vi "PKG_IMC_ClearIMC.vi"(11 "handle":u32) -> (2 "function return":i32, 3 "handle out":u32)   [LabVIEW 2018, in "IMC_Pkg4xxx.lvlib"]
doc: "PKG_IMC_ClearIMC(IMC_HANDLE handle);"
uses:
  IMC_Pkg4xxx.lvlib
  IMC_Pkg4xxx.dll
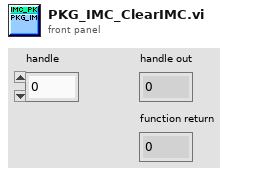
[diagram p1: front panel]
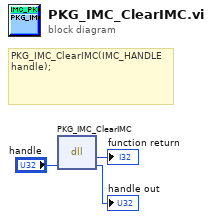
[diagram p0: block diagram]
diagram:
  # "PKG_IMC_ClearIMC(IMC_HANDLE handle);"
  n1 = dll-call lib="PTH2\\abs D做的项目航天测量驱动电机IMCAppincLabview32\nIMC_Pkg4xxx.*" fn="PKG_IMC_ClearIMC"("handle"="handle") -> (→"function return":i32, "handle"=→"handle out":u32)  [unwired: 3 in, 2 out]
